vi "Replace Class References.vi"(8 "error in (no error)":errorcluster, 10 "Target LVClassLibrary ref":refnum<vi>, 11 "vi refnum":refnum<vi>) -> (0 "error out":errorcluster, 2 "Target LVClassLibrary ref out":refnum<vi>)   [LabVIEW 2019, in "gRPC Template Creation Utility.lvlib"]
uses:
  gRPC Template Creation Utility.lvlib
  ServiceConstants.ctl
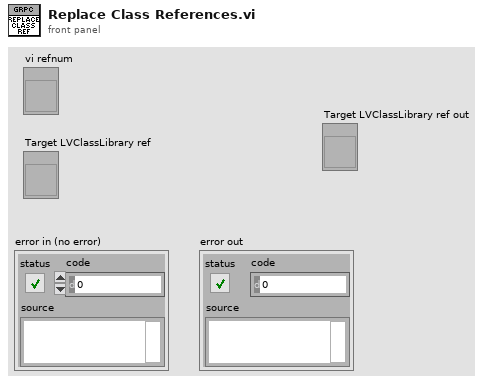
[diagram p1: front panel]
types:
  T1 = typedef "gRPC Template Creation Utility.lvlib/ServiceConstants.ctl" = enum16{"Stub", "Impl", "Usercode_server", "Generated_server", "RPC Service", "RPC Method package_service_method", "ServiceClass out", "ServiceClass in", "RPC Method"}
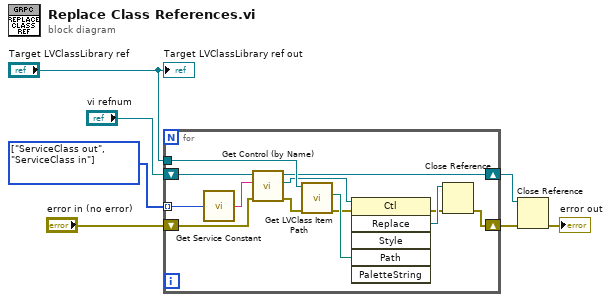
[diagram p0: block diagram]
diagram:
  w7 = T1[] [enum."ServiceClass out", enum."ServiceClass in"] items=["Stub", "Impl", "Usercode_server", "Generated_server", "RPC Service", "RPC Method package_service_method", "ServiceClass out", "ServiceClass in", "RPC Method"]
  n1 = for {
    tunnel: "Target LVClassLibrary ref" -> [w19]
    shift-right: [w10] -> w3
    shift-left: "vi refnum" -> [w17]
    shift-right: [w11] -> w2
    shift-left: "error in (no error)" -> [w15]
    tunnel: w7 -> [w9] mode=indexing
    n2 = call "Get Service Constant.vi"("Service Constant Strings"=w9) -> ("String Value"=w8:string)
    n3 = call "Get Control (by Name).vi"("error in (no error)"=w15, "Control Label"=w8, "Owner VI in"=w17) -> ("error out"=w16:errorcluster, "Control Refnum"=w18:refnum<vi>, "Owner VI out"=w10:refnum<vi>)  [unwired: 5 in, 1 out]
    n4 = call "Get LVClass Item Path.vi"("error in (no error)"=w16, "LVClassLibrary in"=w19) -> ("error out"=w14:errorcluster, "Path"=w20:path)  [unwired: 7 in, 1 out]
    n5 = invoke class="Ctl" method="Replace"(reference=w18, error in=w14, "Path"=w20) -> (error out=w12:errorcluster, "Replace"=w13:refnum<vi>)  [unwired: 3 in, 4 out]
    n6 = Close Reference(reference=w13, error in (no error)=w12) -> (error out=w11:errorcluster)
  }
  n7 = Close Reference(reference=w3, error in (no error)=w2) -> (error out=→"error out":errorcluster)
  "Target LVClassLibrary ref out" <- "Target LVClassLibrary ref"
